vi "Acquire Physical Channels.vi"(8 "error in":errorcluster, 11 "4300 in":refnum<class "4300.lvclass">) -> (0 "error out":errorcluster, 3 "4300 out":refnum<class "4300.lvclass">)   [LabVIEW 2019, in "4300.lvlib" / "4300.lvclass"]
uses:
  Library/4300.lvclass
  C:/Users/Public/Documents/Development/builds/Instruments/Instruments.lvlibp/Library/Instruments.lvclass
  Library/4300.lvclass/4300.ctl
  builds/Instruments/Instruments.lvlibp/Accessors/Read Resource.vi
  <resource>/objmgr/daqmx.rc
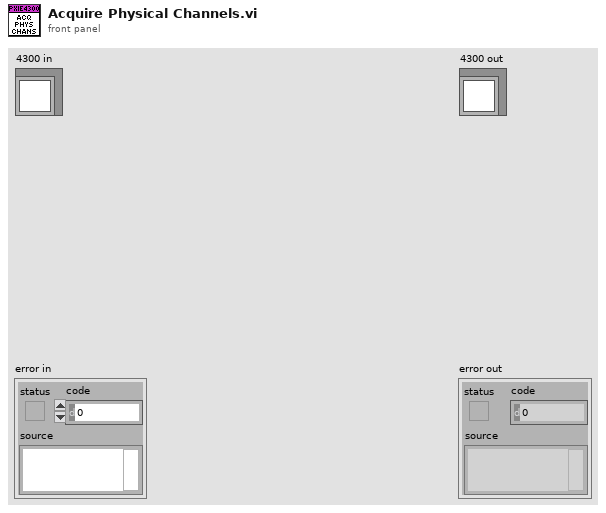
[diagram p1: front panel]
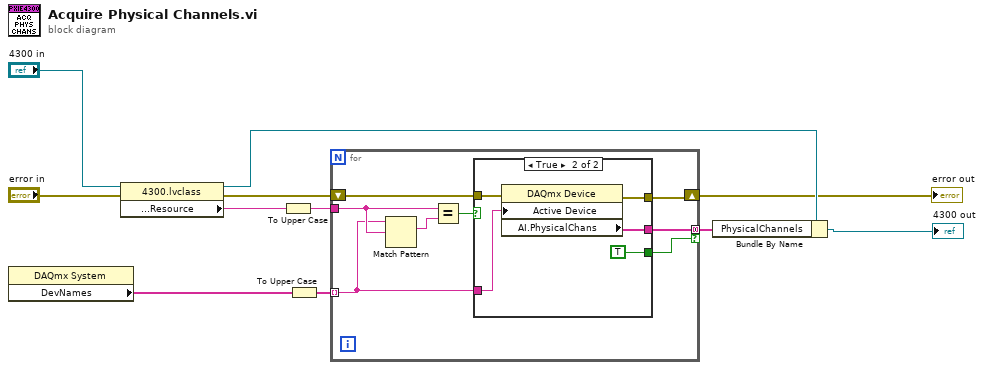
[diagram p0: block diagram]
diagram:
  n1 = property class="DAQmx System"() -> ("DevNames"=w2:tag[])  [unwired: 2 in, 2 out]
  n2 = property class="4300.lvclass"(reference="4300 in", error in="error in") -> (reference out=w8:refnum<class "4300.lvclass">, error out=w4:errorcluster, "Accessors:Configuration:Resource"=w10:string)
  n3 = To Upper Case(1:w10) -> (0:w9:string)
  n4 = To Upper Case(1:w2) -> (0:w1:string[])
  n5 = for {
    tunnel: w1 -> [w12] mode=indexing
    tunnel: w9 -> [w18]
    shift-right: [w16] -> w3
    shift-left: w4 -> [w15]
    tunnel: [w14] -> w6 mode=concatenating if=w13
    # "Find all devices identified as the named resource, list all channels on appropriate analog inputs"
    n6 = Match Pattern(string=w12, regular expression=w18) -> (match substring=w19:string)  [unwired: 1 in, 3 out]
    n7 = Equal?(x=w18, y=w19) -> (x = y?=w17:bool)
    n8 = case shown="True" w17 {
      selector: w17 -> [w20 _]
      tunnel: [w21 w26] -> w16
      tunnel: w15 -> [w21 w25]
      tunnel: w12 -> [_ w24]
      tunnel: [_ w23] -> w14
      tunnel: [w20 TRUE] -> w13
      frame False {
      }
      frame True {
        n9 = property class="DAQmx Device"(error in=w25, "Active Device"=w24) -> (error out=w26:errorcluster, "AI.PhysicalChans"=w23:tag[])  [unwired: 1 in, 1 out]
      }
    }
  }
  "error out" <- w3
  n10 = Bundle By Name(cluster=w8, "PhysicalChannels"=w6) -> (→"4300 out":refnum<class "4300.lvclass">)
